vi "LJM save new configs.vi"(0 "Working Directory":path, 1 "App name":string="LJM_Exp", 2 "Max File Size (Bytes)":i32=1048576, 3 "Write To File":bool, 4 "Disable Scaling":bool, 5 "error in":errorcluster, 6 "Data File Prefix":string="data", 8 "Scan Rate (Hz)":dbl=500.0 format="%.3f", 9 "Interval (ms)":u32=500, 10 "Graph History":i32=1000 min=0, 11 "Resolution":u8, 12 "# Channels":i32=4, 13 "SettlingFactor":u8, 17 "Channel Setup":T1={"+Ch"=["0", "1", "2", "3", "4", "5", "6", "7"], "-Ch"=["199", "199", "199", "199", "199", "199", "199", "199"], "Ranges"=[0, 0, 0, 0, 0, 0, 0, 0], "Scaling Equation"=["y=v0", "y=v1", "y=v2", "y=v3", "y=v4", "y=v5", "y=v6", "y=v7"], "Graph?"=[]} {"Ranges" items=["LJ_rgBIP10V", "LJ_rgBIP5V", "LJ_rgUNI5V", "LJ_rgUNI2P5V", "LJ_rgUNI1P25V", "LJ_rgBIP1V", "LJ_rgUNIP625V", "LJ_rgBIPP1V", "LJ_rgBIPP01V"]}) -> (14 "Working Directory Out":path, 19 "error out":errorcluster)   [LabVIEW 2022 SP3]
uses:
  Instance           1 28Saved   LJM save new configs .vi
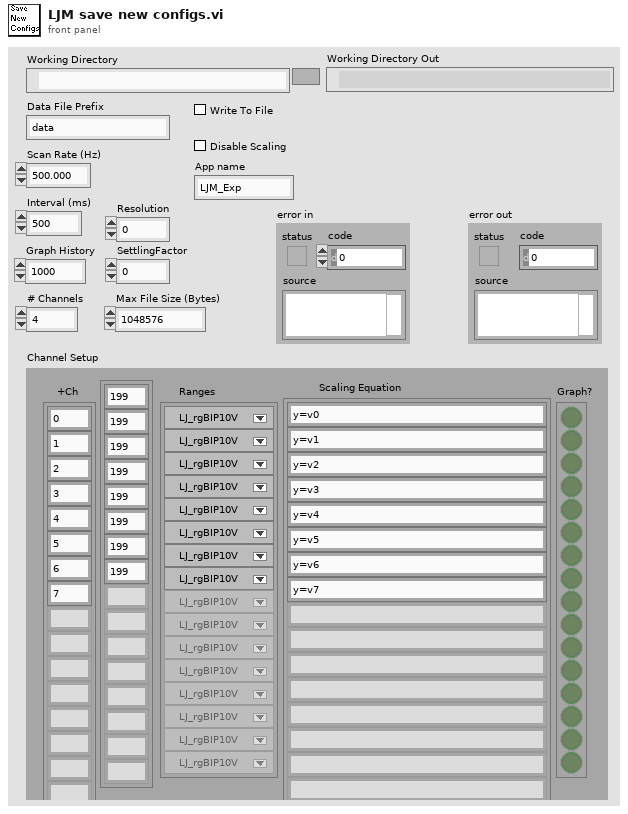
[diagram p1: front panel]
types:
  T1 = cluster{"+Ch":string[], "-Ch":string[], "Ranges":u16[], "Scaling Equation":string[], "Graph?":bool[]}
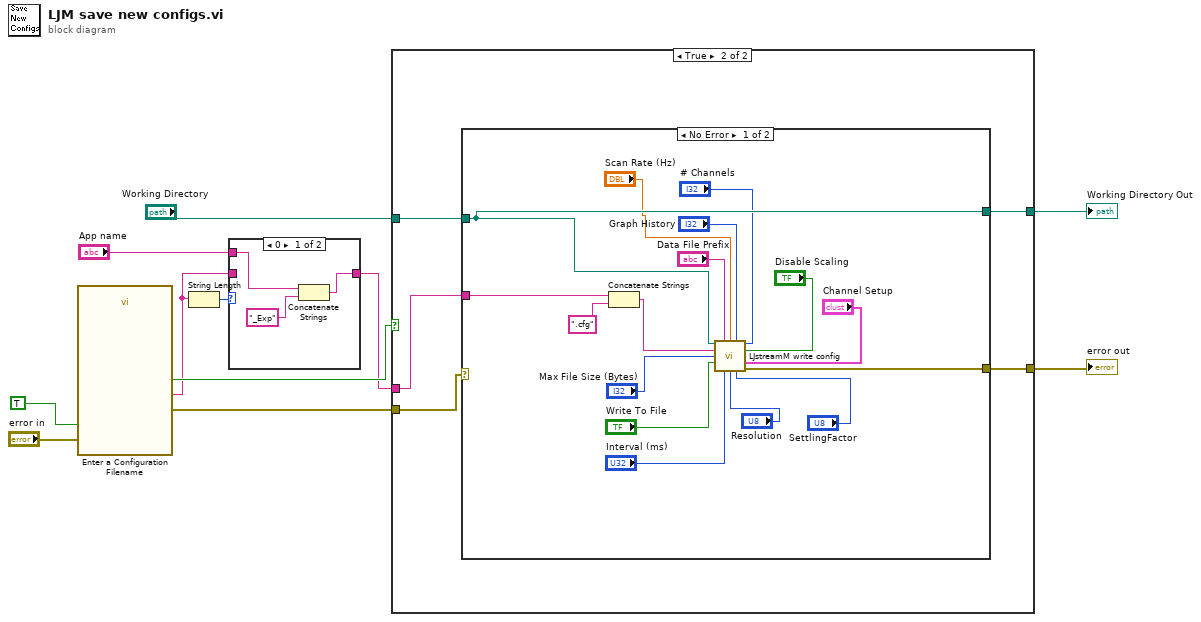
[diagram p0: block diagram]
diagram:
  n1 = call "Enter a Configuration Filename"("Enable"=TRUE, "error in (no error)"="error in") -> ("Filename"=w3:string, "OK"=w5:bool, "error out"=w6:errorcluster)  [unwired: 15 in]
  n2 = String Length(string=w3) -> (length=w4:i32)
  n3 = case shown="0" w4 {
    tunnel: w3 -> [_ w15]
    tunnel: [w12 w15] -> w2
    tunnel: "App name" -> [w14 _]
    frame 0 {
      n4 = Concatenate Strings(w14, "_Exp" ("string")) -> (w12:string)
    }
    frame 1, Default {
    }
  }
  n5 = case shown="True" w5 {
    tunnel: [w16 w22] -> w11
    tunnel: [w17 w21] -> w10
    tunnel: "Working Directory" -> [w17 w20]
    tunnel: w2 -> [_ w19]
    tunnel: w6 -> [w16 w18]
    frame False {
    }
    frame True {
      n6 = case shown="No Error" w18 {
        selector: w18 -> [_ w40]
        tunnel: [w37 w40] -> w22
        tunnel: [w38 w39] -> w21
        tunnel: w20 -> [w38 w39]
        tunnel: w19 -> [w24 _]
        frame No Error {
          n7 = Concatenate Strings(w24, ".cfg" ("string")) -> (w33:string)
          n8 = call "LJstreamM write config.vi"("Working Directory"=w38, "Data File Prefix"="Data File Prefix", "Scan Rate (Hz)"="Scan Rate (Hz)", "Graph History"="Graph History", "# Channels"="# Channels", "filename"=w33, "Disable Scaling"="Disable Scaling", "Max File Size (Bytes)"="Max File Size (Bytes)", "Write To File"="Write To File", "Channel Setup"="Channel Setup", "Interval (ms)"="Interval (ms)", "Resolution"="Resolution", "SettlingFactor"="SettlingFactor") -> ("error out"=w37:errorcluster)  [unwired: 2 in]
        }
        frame Error {
        }
      }
    }
  }
  "error out" <- w11
  "Working Directory Out" <- w10
